vi "Timing Source Initialization.vi"(8 "error in (no error)":errorcluster, 10 "Loop Time (usec)":u32, 11 "Device Ref":T1=18446744073709551615 format="%.0x") -> (0 "error out":errorcluster, 1 "Primary Control Loop dt":i64, 2 "Actual Loop Rate (Hz)":dbl, 3 "Timing Source Name":string, 4 "Do not destroy the custom timing source":bool)   [LabVIEW 2019, in "TelemetryAsync Engine.lvlib"]
uses:
  TelemetryAsync Engine.lvlib
  <vilib>/NI VeriStand/Custom Device API/Custom Device Item Ref.ctl
  <vilib>/Platform/TimedLoop/scheduler/LVUserAPI/_suppVIs/Create_1kHz_TSource.vi
  <vilib>/NI VeriStand/Custom Device API/Custom Device API.lvlib
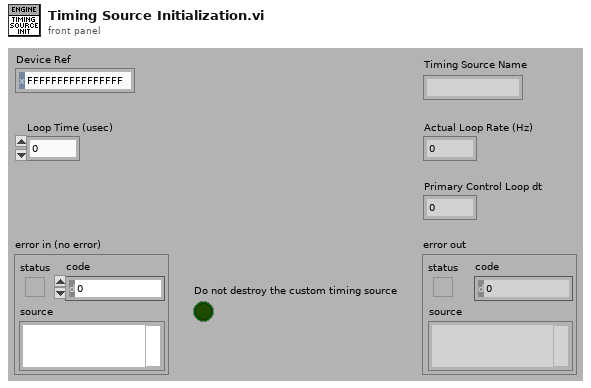
[diagram p1: front panel]
types:
  T1 = typedef "Custom Device API.lvlib/Custom Device Item Ref.ctl" = u64
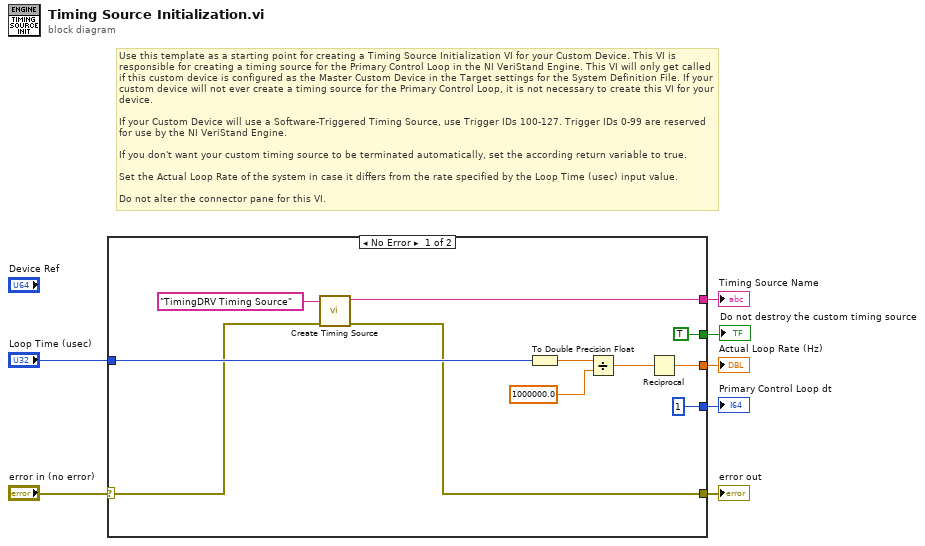
[diagram p0: block diagram]
diagram:
  # "Use this template as a starting point for creating a Timing Source Initialization VI for your Custom Device. This VI is responsible for creating a timing source for the Primary Control Loop in the NI VeriStand Engine. This VI will only get called if this custom device is configured as the Master Custom Device in the Target settings for the System Definition File. If your custom device will not ever create a timing source for the Primary Control Loop, it is not necessary to create this VI for your device.\n\nIf your Custom Device will use a Software-Triggered Timing Source, use Trigger IDs 100-127. Trigger IDs 0-99 are reserved for use by the NI VeriStand Engine.\n\nIf you don't want your custom timing source to be terminated automatically, set the according return variable to true.\n\nSet the Actual Loop Rate of the system in case it differs from the rate specified by the Loop Time (usec) input value.\n\nDo not alter the connector pane for this VI."
  n1 = case shown="No Error" "error in (no error)" {
    selector: "error in (no error)" -> [w9 w19]
    tunnel: [w8 w19] -> w7
    tunnel: "Loop Time (usec)" -> [w18 _]
    tunnel: [w14 _] -> w4
    tunnel: [w12 _] -> w3
    tunnel: [i64 1 ("Primary Control Loop dt") _] -> w2
    tunnel: [TRUE ("Do not destroy the custom timing source") _] -> w1
    frame No Error {
      n2 = call-poly <vilib>:"Create Timing Source.vi"("error in (no error)"=w9, "name (in)"="TimingDRV Timing Source") -> ("error out"=w8:errorcluster, "name (out)"=w12:string)  [unwired: 8 in]
      n3 = To Double Precision Float(number=w18) -> (double precision float=w17:dbl)
      n4 = Divide(x=w17, y=1000000.0) -> (x/y=w15:dbl)
      n5 = Reciprocal(x=w15) -> (1/x=w14:dbl)
    }
    frame Error {
    }
  }
  "error out" <- w7
  "Timing Source Name" <- w3
  "Actual Loop Rate (Hz)" <- w4
  "Primary Control Loop dt" <- w2
  "Do not destroy the custom timing source" <- w1
